vi "Get Inset Image JPG Path.vi"(4 "Inset Data Path":path, 5 "Inkscape Path":path) -> (1 "Inset JPG Path":path)   [LabVIEW 2019]
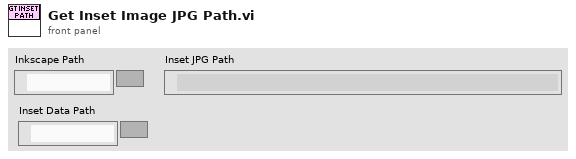
[diagram p1: front panel]
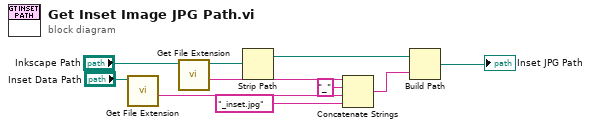
[diagram p0: block diagram]
diagram:
  n1 = call <vilib>:"Get File Extension.vi"("file"="Inset Data Path") -> ("filename without extension"=w2:string)  [unwired: 6 in, 4 out]
  n2 = call <vilib>:"Get File Extension.vi"("file"="Inkscape Path") -> ("filename without extension"=w8:string, "dup file"=w9:path)  [unwired: 6 in, 3 out]
  n3 = Strip Path(path=w9) -> (stripped path=w6:path)  [unwired: 1 out]
  n4 = Concatenate Strings(w8, "_" ("string"), w2, "_inset.jpg" ("string")) -> (w5:string)
  n5 = Build Path(base path=w6, name or relative path=w5) -> (appended path=→"Inset JPG Path":path)
